vi "Laser.vi"(8 "error in (no error)":errorcluster, 10 "Notifiers":T1, 11 "All Message Queue Cluster":T2) -> (0 "error out":errorcluster)   [LabVIEW 2017]
doc: "Ce VI est la partie visualisation du Laser"
uses:
  Lib QMH/AllMessageQueue Cluster.ctl
  Lib QMH/Message Cluster.ctl
  Lib Notifier/Notifier.ctl
  Laser UI data.ctl
  PulsePickerValues.ctl
  Laser config.ctl
  FGV Laser/Action Laser.ctl
  FGV Laser/FGV Laser Data.ctl
  Lib IHM Control/Front Panel Status.ctl
  support/Status.vi
  Lib QMH/MessageQueues.lvlib
  Lib IHM Control/IHM Control.lvlib
  Lib Notifier/Notifier.lvlib
panel:
  out "Pulse Picker":dbl format="%#_3g"
  out "Power":dbl format="%#_3g"
  out "Connected":bool
  out "Status":string
  # "Laser"
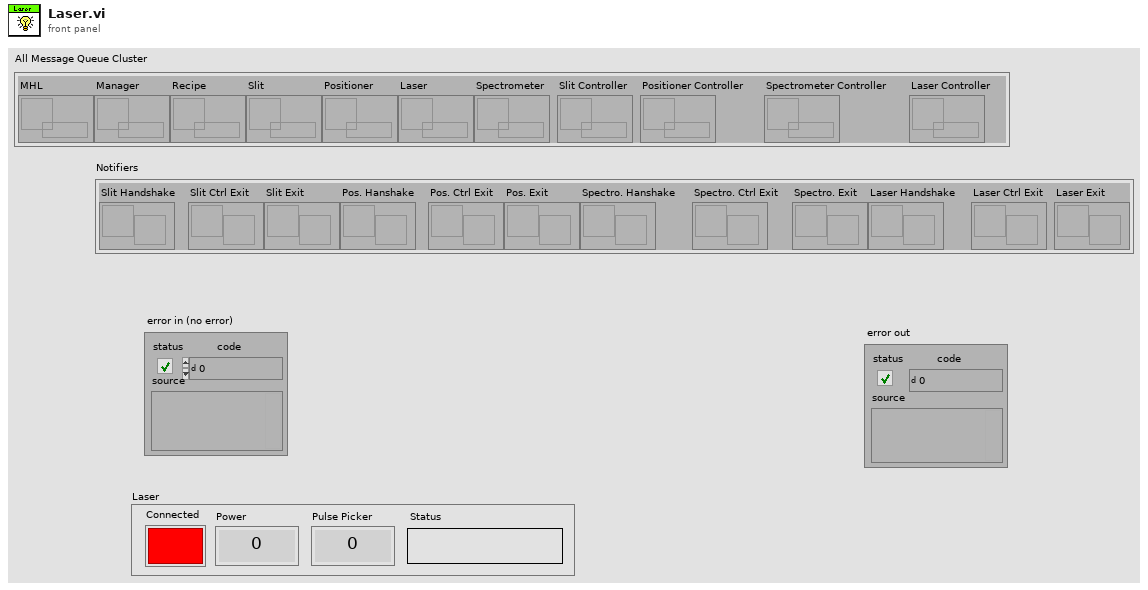
[diagram p1: front panel]
types:
  T1 = typedef "Notifier.lvlib/Notifier.ctl" = cluster{"Slit Handshake":refnum<notifier>, "Slit Ctrl Exit":refnum<notifier>, "Slit Exit":refnum<notifier>, "Pos. Hanshake":refnum<notifier>, "Pos. Ctrl Exit":refnum<notifier>, "Pos. Exit":refnum<notifier>, "Spectro. Hanshake":refnum<notifier>, "Spectro. Ctrl Exit":refnum<notifier>, "Spectro. Exit":refnum<notifier>, "Laser Handshake":refnum<notifier>, "Laser Ctrl Exit":refnum<notifier>, "Laser Exit":refnum<notifier>}
  T2 = typedef "MessageQueues.lvlib/AllMessageQueue Cluster.ctl" = cluster{"MHL":refnum<queue>, "Manager":refnum<queue>, "Recipe":refnum<queue>, "Slit":refnum<queue>, "Positioner":refnum<queue>, "Laser":refnum<queue>, "Spectrometer":refnum<queue>, "Slit Controller":refnum<queue>, "Positioner Controller":refnum<queue>, "Spectrometer Controller":refnum<queue>, "Laser Controller":refnum<queue>}
  T3 = typedef "FGV Laser Data.ctl" = cluster{"ONLINE":bool, "Power":dbl, "VISA resource name out":refnum<visa-resource-name>, "Time Out":dbl, "Status":string, "Read Count":u32, "On/OFF":bool, "Pulse Picker Set":T4}
  T4 = typedef "PulsePickerValues.ctl" = u16
  T5 = typedef "Action Laser.ctl" = enum16{"Initialize", "Connect", "Disconnect", "Set Power", "Get Power", "Set Pulse Picker", "Get Pulse Picker", "Laser ON", "Laser OFF", "Read Visa"}
  T6 = typedef "IHM Control.lvlib/Front Panel Status.ctl" = enum16{"Initialisation", "Enable Slit", "Enable Positionner", "Enable Spectrometer", "Enable Laser", "Disable Slit", "Disable Positionner", "Disable Spectrometer", "Disable Laser"}
  T7 = typedef "Laser config.ctl" = cluster{"VISA resource name":refnum<visa-resource-name>}
  T8 = typedef "Laser UI data.ctl" = cluster{"Connected":bool, "Status":string, "Power":dbl, "Pulse Picker Set":T4}
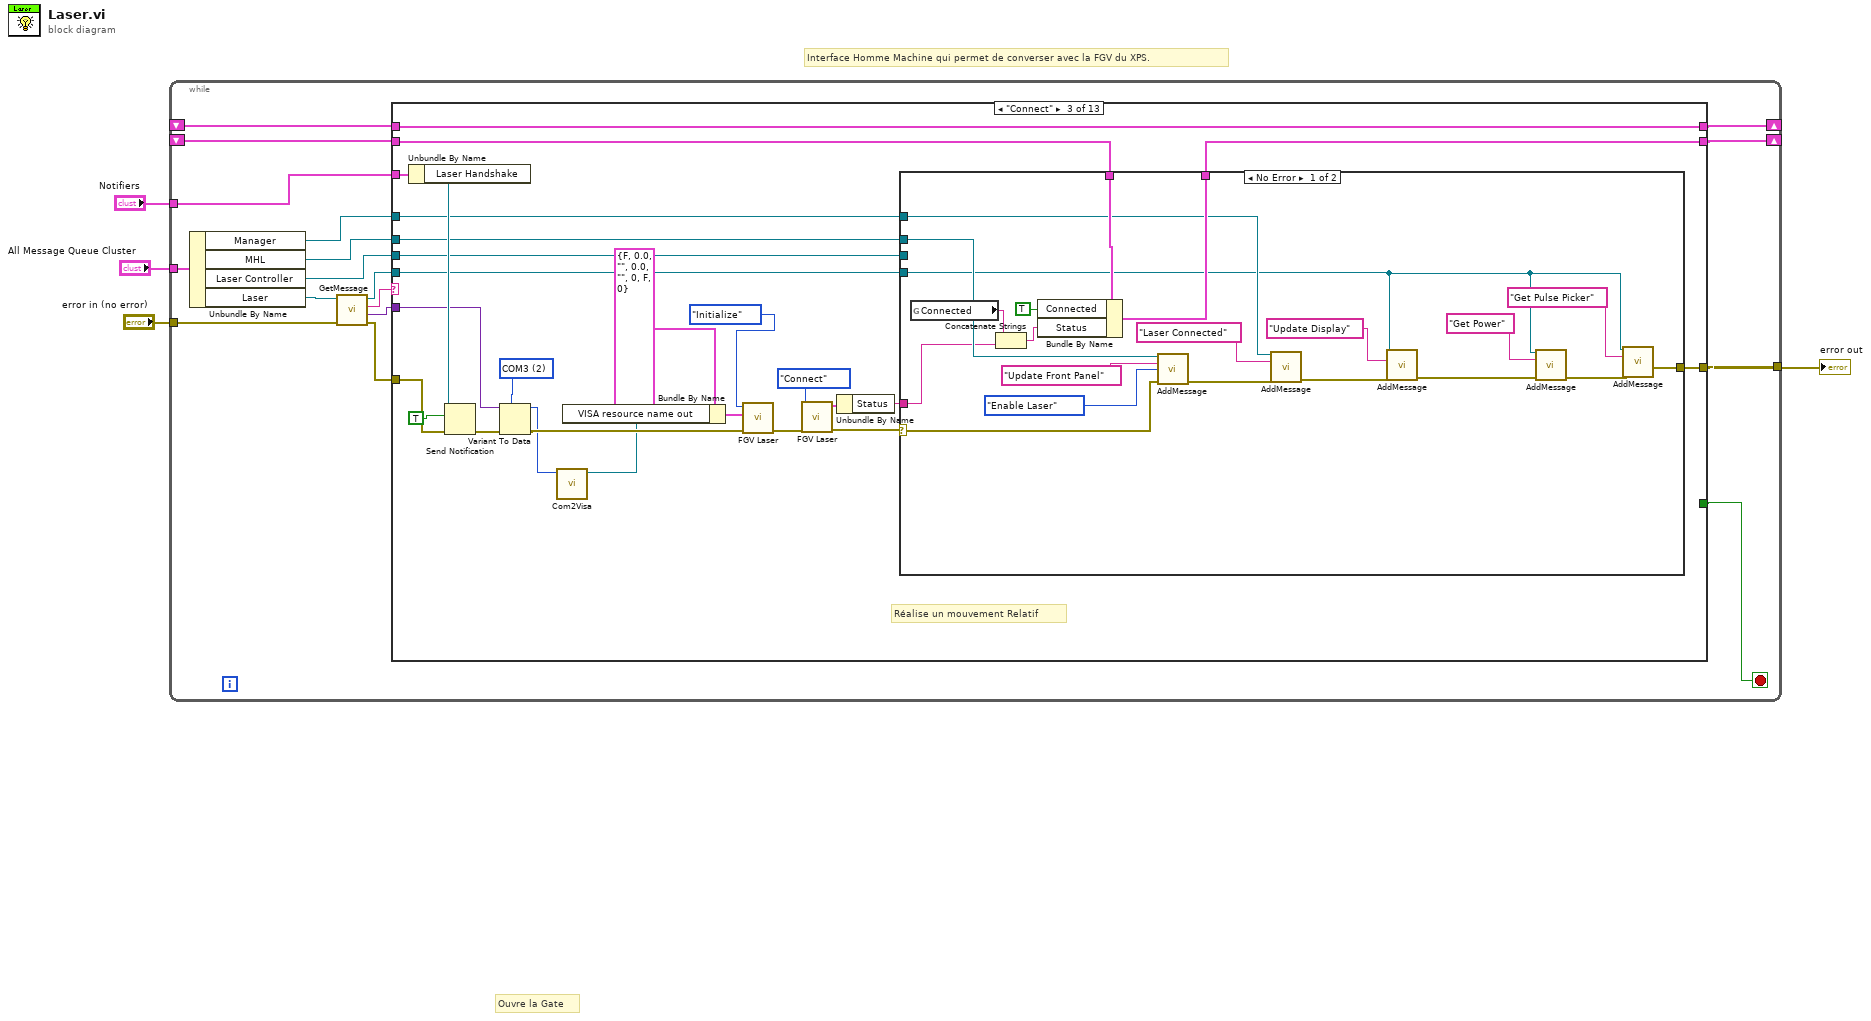
[diagram p0: block diagram]
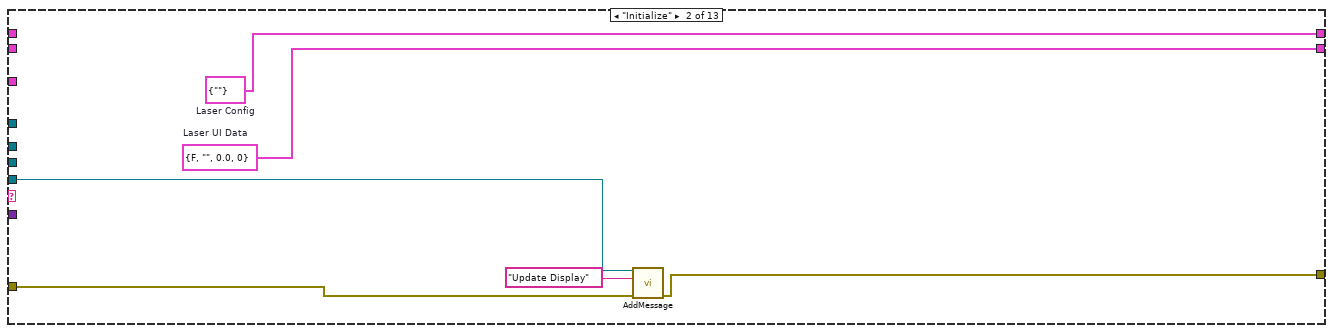
[diagram p3: hidden frame]
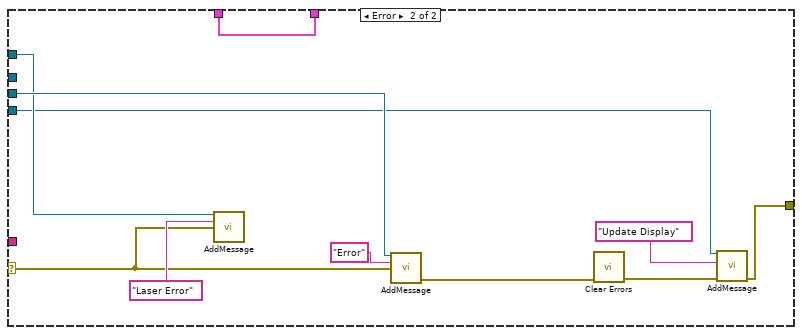
[diagram p4: hidden frame]
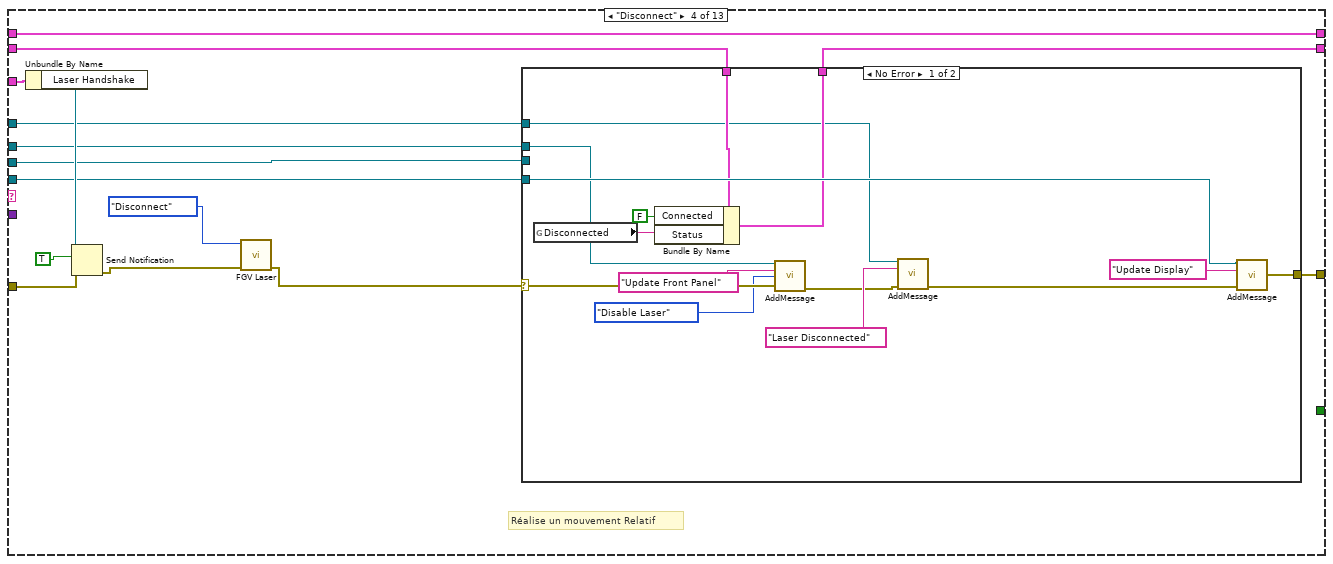
[diagram p5: hidden frame]
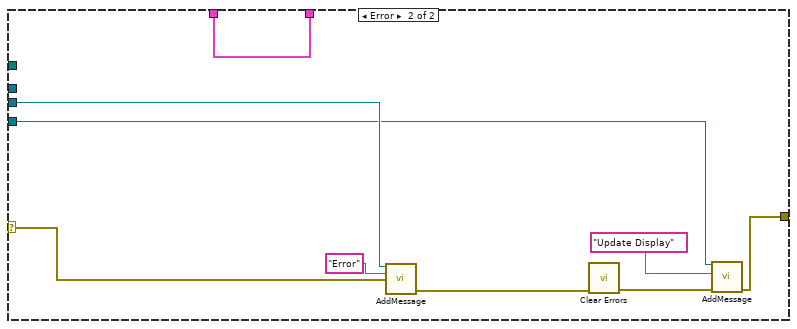
[diagram p6: hidden frame]
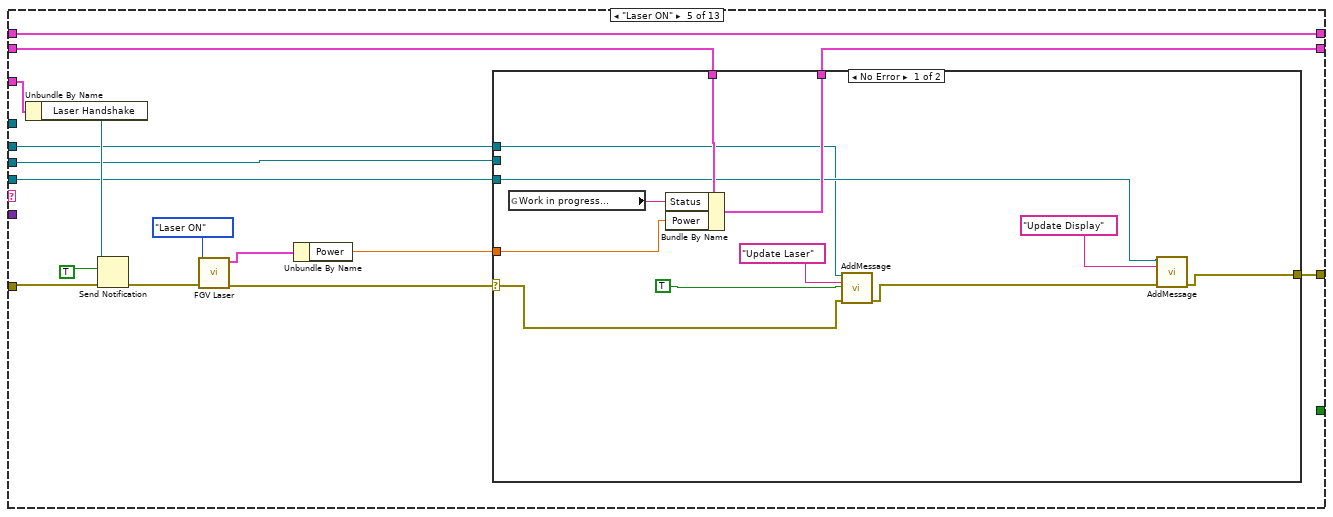
[diagram p7: hidden frame]
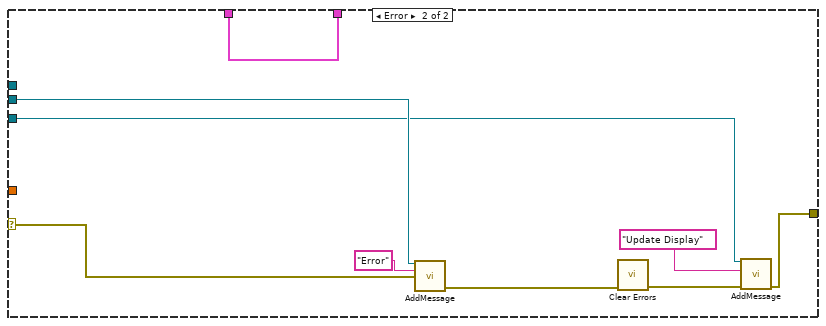
[diagram p8: hidden frame]
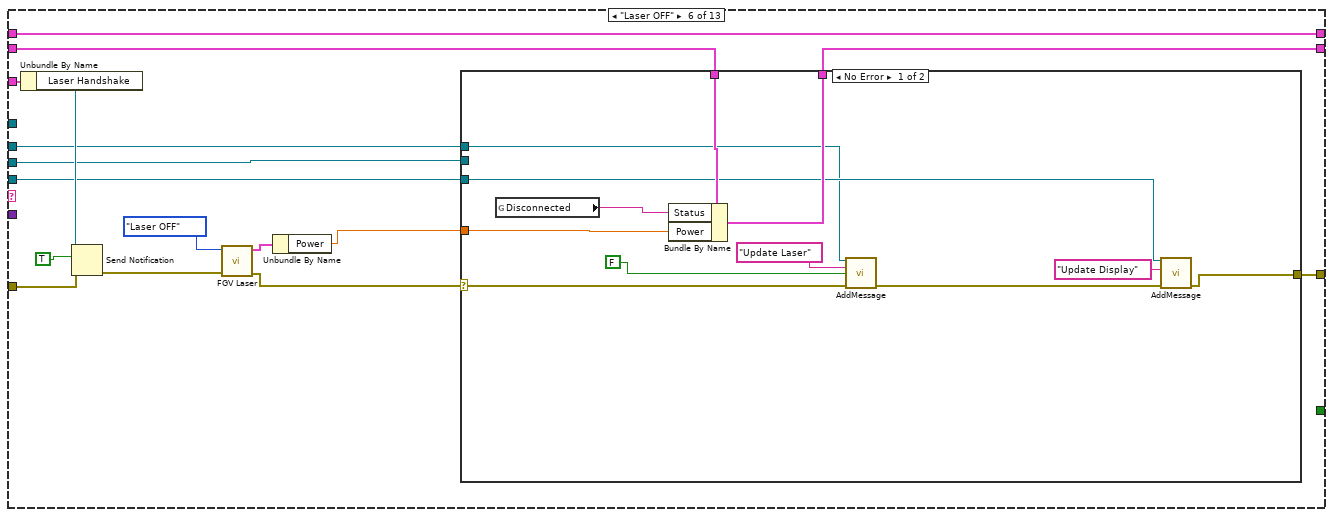
[diagram p9: hidden frame]
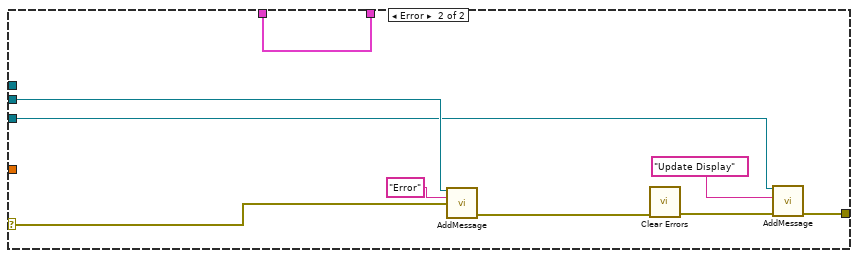
[diagram p10: hidden frame]
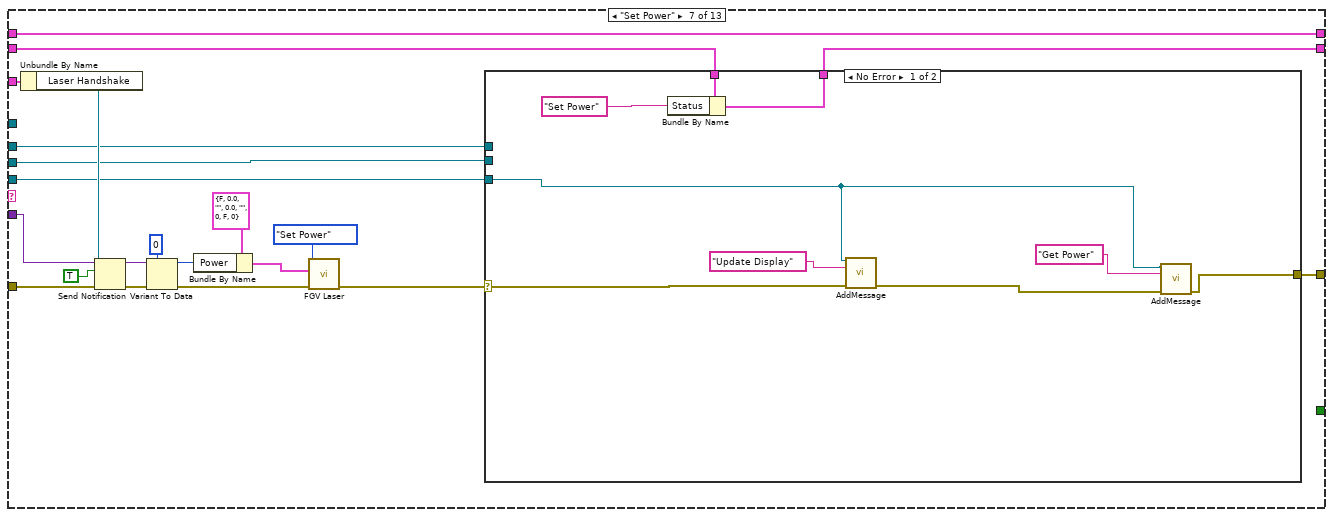
[diagram p11: hidden frame]
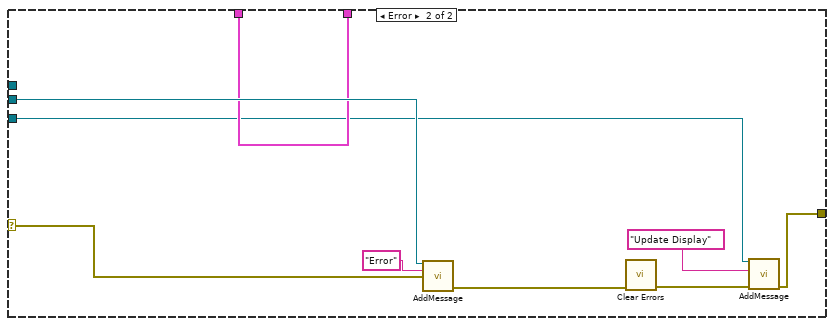
[diagram p12: hidden frame]
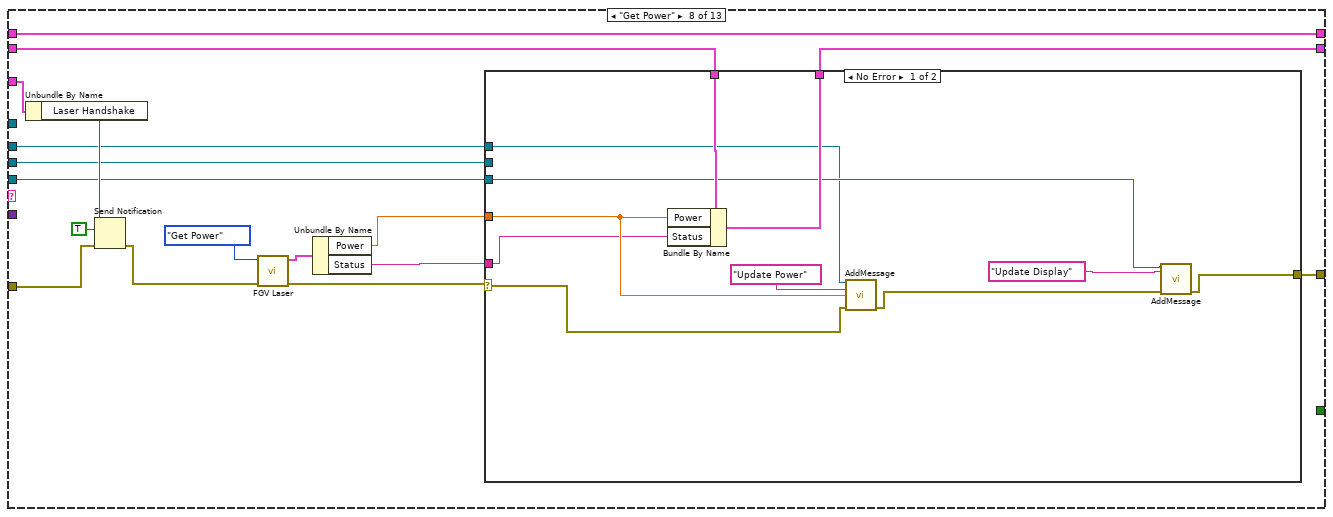
[diagram p13: hidden frame]
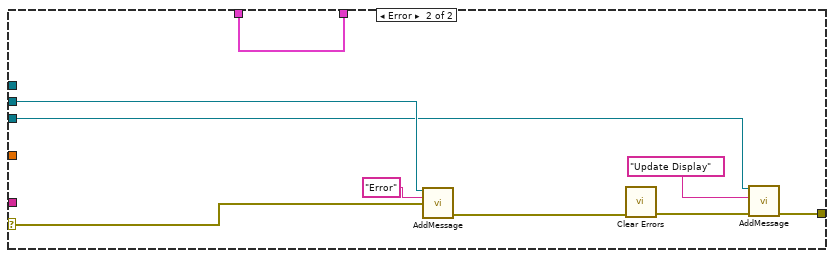
[diagram p14: hidden frame]
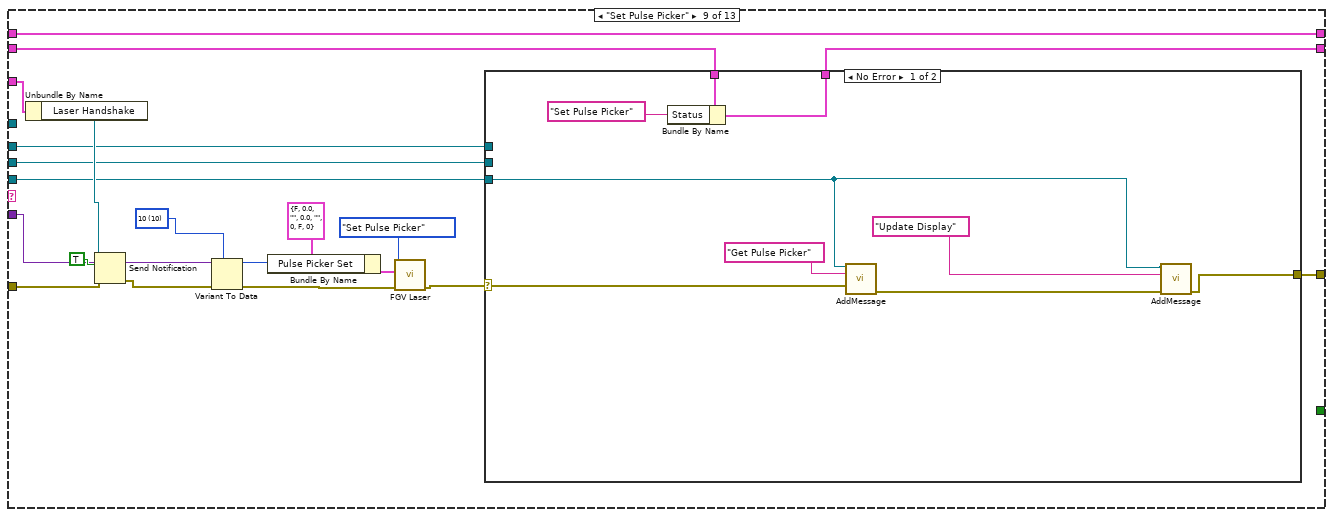
[diagram p15: hidden frame]
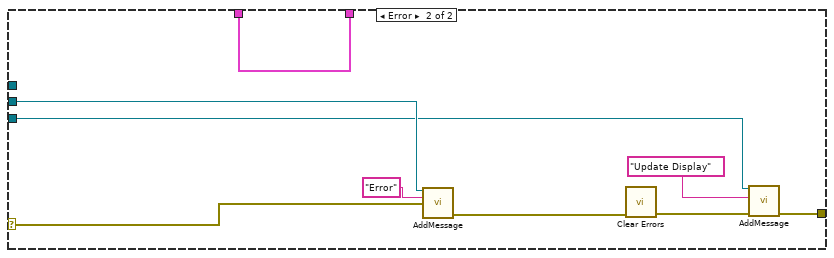
[diagram p16: hidden frame]
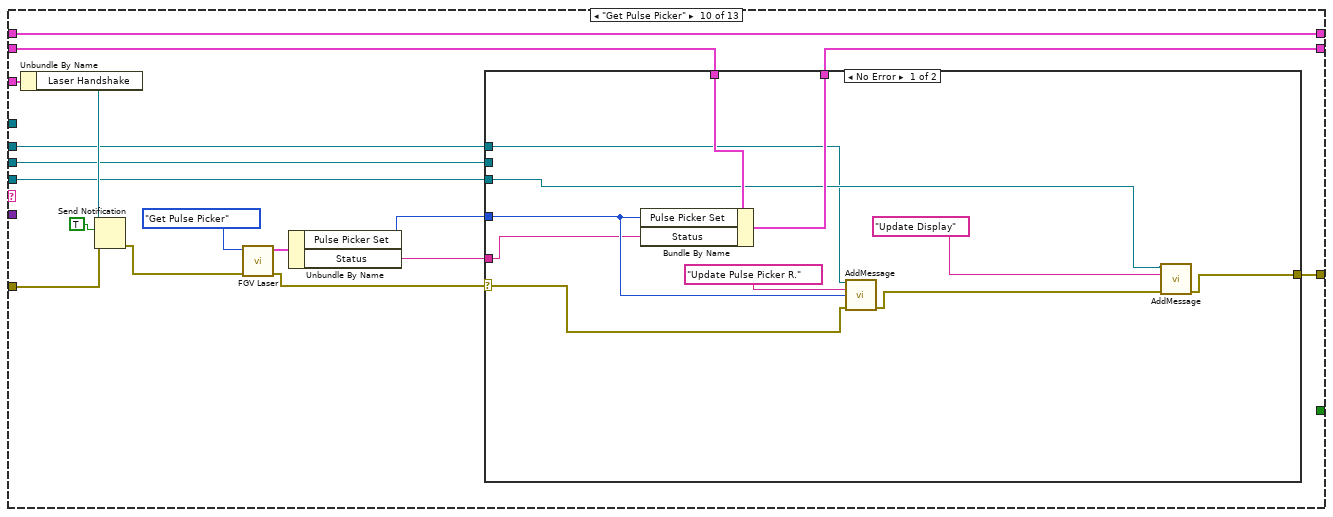
[diagram p17: hidden frame]
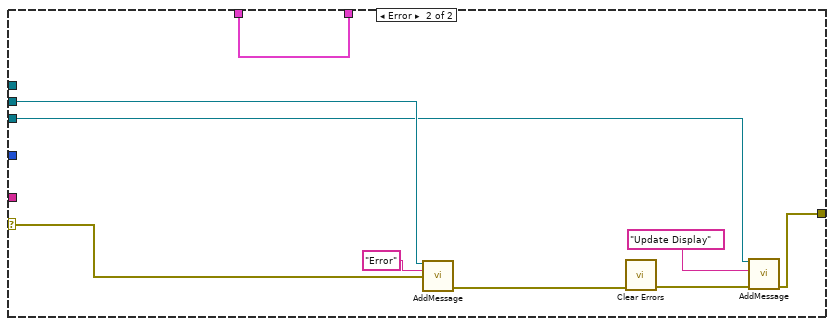
[diagram p18: hidden frame]
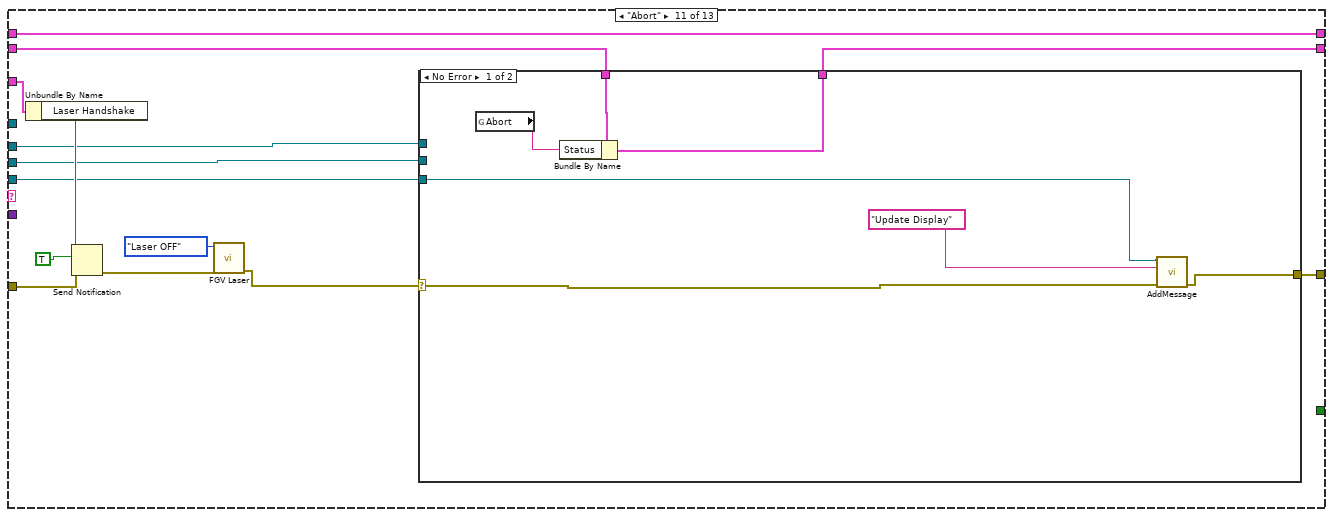
[diagram p19: hidden frame]
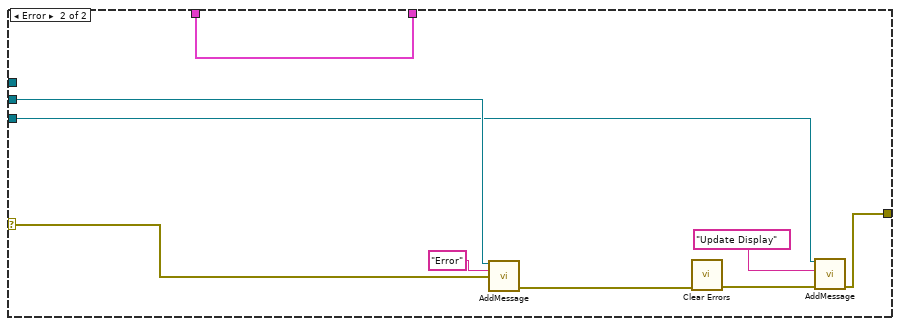
[diagram p20: hidden frame]
diagram:
  # "Interface Homme Machine qui permet de converser avec la FGV du XPS."
  # "Ouvre la Gate"
  n1 = while {
    tunnel: "All Message Queue Cluster" -> [w19]
    tunnel: "Notifiers" -> [w12]
    tunnel: "error in (no error)" -> [w20]
    tunnel: [w14] -> w1
    shift-right: [w16] -> _
    shift-left: _ -> [w18]
    shift-right: [w15] -> _
    shift-left: _ -> [w17]
    stop <- w13 stop-if-true
    n2 = Unbundle By Name(w19) -> ("Manager"=w11:refnum<queue>, "MHL"=w10:refnum<queue>, "Laser Controller"=w9:refnum<queue>, "Laser"=w21:refnum<queue>)
    n3 = call "GetMessage.vi"("entrée d'erreur"=w20, "Message queue"=w21) -> ("sortie d'erreur"=w7:errorcluster, "Data"=w6:variant, "Message"=w5:string, "Dup Message Queue"=w8:refnum<queue>)  [unwired: 6 in]
    n4 = case shown="\"Connect\"" w5 {
      tunnel: w12 -> [_ _ w54 w101 w141 w178 w219 w254 w294 w329 w363 _ w398]
      tunnel: w8 -> [_ w27 w53 w100 w140 w177 w218 w253 w293 w328 w362 _ w392]
      tunnel: w6 -> [_ _ w43 _ _ _ w211 _ w286 _ _ _ _]
      tunnel: w7 -> [w24 w29 w47 w94 w135 w172 w209 w246 w285 w321 w357 w387 w393]
      tunnel: [w24 w28 w52 w99 w139 w176 w217 w252 w292 w327 w361 w387 w395] -> w14
      tunnel: w9 -> [_ _ w51 w98 w138 w175 w216 w251 w291 w326 w360 _ _]
      tunnel: [_ _ _ _ _ _ _ _ _ _ _ _ TRUE] -> w13
      tunnel: w18 -> [w23 _ w50 w97 w137 w174 w215 w250 w290 w325 w359 w388 w394]
      tunnel: [w23 w26 w50 w97 w137 w174 w215 w250 w290 w325 w359 w388 w394] -> w16
      tunnel: w17 -> [w22 _ w49 w96 w133 w170 w212 w247 w287 w322 w355 w386 w391]
      tunnel: [w22 w25 w48 w95 w136 w173 w214 w249 w289 w324 w358 w386 w391] -> w15
      tunnel: w10 -> [_ _ w46 w93 w134 w171 w213 w248 w288 w323 w356 _ _]
      tunnel: w11 -> [_ _ w45 w92 _ _ _ _ _ _ _ _ _]
      frame Default {
        # "ne fait rien si le message dépilé n'existe pas"
      }
      frame "Initialize" {
        w26 = T7 {"VISA resource name"=""}  # Laser Config
        w25 = T8 {"Connected"=FALSE, "Status"="", "Power"=0.0, "Pulse Picker Set"=0}  # Laser UI Data
        n5 = call "AddMessage.vi"("Message queue"=w27, "Message"="Update Display", "entrée d'erreur (pas d'erreur)"=w29) -> ("error out"=w28:errorcluster)  [unwired: 11 in, 1 out]
      }
      frame "Connect" {
        w33 = 2 items=["COM1", "COM2", "COM3", "COM4", "COM5", "COM6", "COM7", "COM8", "COM9", "COM10", "COM11", "COM12", "COM13", "COM14", "COM15", "COM16", "COM17", "COM18", "COM19", "COM20", "COM21", "COM22", "COM23", "COM24", "COM25", "COM26", "COM27", "COM28", "COM29", "COM30"] ("Portnumber")
        # "Réalise un mouvement Relatif"
        n6 = Unbundle By Name(w54) -> ("Laser Handshake"=w56:refnum<notifier>)
        n7 = Send Notification(notification=TRUE, notifier=w56, error in (no error)=w47) -> (error out=w44:errorcluster)  [unwired: 1 out]
        n8 = Variant To Data(error in=w44, type=w33, Variant=w43) -> (data=w32:i32, error out=w37:errorcluster)
        n9 = call "Com2Visa.vi"("Portnumber"=w32) -> ("VISA Refnum out"=w31:refnum<visa-resource-name>)  [unwired: 10 in]
        n10 = Bundle By Name(cluster=T3 {"ONLINE"=FALSE, "Power"=0.0, "VISA resource name out"="", "Time Out"=0.0, "Status"="", "Read Count"=0, "On/OFF"=FALSE, "Pulse Picker Set"=0} ("FGV Laser Data In"), "VISA resource name out"=w31) -> (w38:T3)
        n11 = call "FGV Laser.vi"("error in (no error)"=w37, "FGV Laser Data In"=w38, "Action"=Action_Laser."Initialize") -> ("error out"=w40:errorcluster)  [unwired: 7 in, 1 out]
        n12 = call "FGV Laser.vi"("error in (no error)"=w40, "Action"=Action_Laser."Connect") -> ("error out"=w36:errorcluster, "FGV Laser Data Out"=w35:T3)  [unwired: 8 in]
        n13 = Unbundle By Name(w35) -> ("Status"=w34:string)
        n14 = case shown="No Error" w36 {
          selector: w36 -> [w73 w79]
          tunnel: w53 -> [w58 w78]
          tunnel: [w60 w84] -> w52
          tunnel: w51 -> [_ w83]
          tunnel: w49 -> [w76 w82]
          tunnel: [w75 w82] -> w48
          tunnel: w46 -> [w72 _]
          tunnel: w45 -> [w67 w80]
          tunnel: w34 -> [w63 _]
          frame No Error {
            n15 = global read "Status.vi" "Connected"() -> (w65:string)
            n16 = Concatenate Strings(w65, w63) -> (w64:string)
            n17 = Bundle By Name(cluster=w76, "Connected"=TRUE, "Status"=w64) -> (w75:T8)
            n18 = call "AddMessage.vi"("Message queue"=w72, "Message"="Update Front Panel", "Data"=Front_Panel_Status."Enable Laser" ("Front Panel status"), "entrée d'erreur (pas d'erreur)"=w73) -> ("error out"=w69:errorcluster)  [unwired: 10 in, 1 out]
            n19 = call "AddMessage.vi"("Message queue"=w67, "Message"="Laser Connected", "entrée d'erreur (pas d'erreur)"=w69) -> ("error out"=w68:errorcluster)  [unwired: 11 in, 1 out]
            n20 = call "AddMessage.vi"("Message queue"=w58, "Message"="Update Display", "entrée d'erreur (pas d'erreur)"=w68) -> ("error out"=w62:errorcluster)  [unwired: 11 in, 1 out]
            n21 = call "AddMessage.vi"("Message queue"=w58, "Message"="Get Power", "entrée d'erreur (pas d'erreur)"=w62) -> ("error out"=w61:errorcluster)  [unwired: 11 in, 1 out]
            n22 = call "AddMessage.vi"("Message queue"=w58, "Message"="Get Pulse Picker", "entrée d'erreur (pas d'erreur)"=w61) -> ("error out"=w60:errorcluster)  [unwired: 11 in, 1 out]
          }
          frame Error {
            n23 = call "AddMessage.vi"("Message queue"=w80, "Message"="Laser Error", "Data"=w79) -> ()  [unwired: 11 in, 2 out]
            n24 = call "AddMessage.vi"("Message queue"=w83, "Message"="Error", "Data"=w79) -> ("error out"=w87:errorcluster)  [unwired: 11 in, 1 out]
            n25 = call <vilib>:"Clear Errors.vi"("error in (no error)"=w87) -> ("error out"=w85:errorcluster)  [unwired: 5 in, 1 out]
            n26 = call "AddMessage.vi"("Message queue"=w78, "Message"="Update Display", "entrée d'erreur (pas d'erreur)"=w85) -> ("error out"=w84:errorcluster)  [unwired: 11 in, 1 out]
          }
        }
      }
      frame "Disconnect" {
        # "Réalise un mouvement Relatif"
        n27 = Unbundle By Name(w101) -> ("Laser Handshake"=w103:refnum<notifier>)
        n28 = Send Notification(notification=TRUE, notifier=w103, error in (no error)=w94) -> (error out=w91:errorcluster)  [unwired: 1 out]
        n29 = call "FGV Laser.vi"("error in (no error)"=w91, "Action"=Action_Laser."Disconnect") -> ("error out"=w90:errorcluster)  [unwired: 8 in, 1 out]
        n30 = case shown="No Error" w90 {
          selector: w90 -> [w112 w122]
          tunnel: w100 -> [w118 w119]
          tunnel: [w116 w123] -> w99
          tunnel: w98 -> [_ w121]
          tunnel: w96 -> [w115 w120]
          tunnel: [w114 w120] -> w95
          tunnel: w93 -> [w111 _]
          tunnel: w92 -> [w105 _]
          frame No Error {
            n31 = global read "Status.vi" "Disconnected"() -> (w104:string)
            n32 = Bundle By Name(cluster=w115, "Connected"=FALSE, "Status"=w104) -> (w114:T8)
            n33 = call "AddMessage.vi"("Message queue"=w111, "Message"="Update Front Panel", "Data"=Front_Panel_Status."Disable Laser" ("Front Panel status"), "entrée d'erreur (pas d'erreur)"=w112) -> ("error out"=w107:errorcluster)  [unwired: 10 in, 1 out]
            n34 = call "AddMessage.vi"("Message queue"=w105, "Message"="Laser Disconnected", "entrée d'erreur (pas d'erreur)"=w107) -> ("error out"=w106:errorcluster)  [unwired: 11 in, 1 out]
            n35 = call "AddMessage.vi"("Message queue"=w118, "Message"="Update Display", "entrée d'erreur (pas d'erreur)"=w106) -> ("error out"=w116:errorcluster)  [unwired: 11 in, 1 out]
          }
          frame Error {
            n36 = call "AddMessage.vi"("Message queue"=w121, "Message"="Error", "Data"=w122) -> ("error out"=w126:errorcluster)  [unwired: 11 in, 1 out]
            n37 = call <vilib>:"Clear Errors.vi"("error in (no error)"=w126) -> ("error out"=w124:errorcluster)  [unwired: 5 in, 1 out]
            n38 = call "AddMessage.vi"("Message queue"=w119, "Message"="Update Display", "entrée d'erreur (pas d'erreur)"=w124) -> ("error out"=w123:errorcluster)  [unwired: 11 in, 1 out]
          }
        }
      }
      frame "Laser ON" {
        n39 = Unbundle By Name(w141) -> ("Laser Handshake"=w143:refnum<notifier>)
        n40 = Send Notification(notification=TRUE, notifier=w143, error in (no error)=w135) -> (error out=w132:errorcluster)  [unwired: 1 out]
        n41 = call "FGV Laser.vi"("error in (no error)"=w132, "Action"=Action_Laser."Laser ON") -> ("error out"=w131:errorcluster, "FGV Laser Data Out"=w129:T3)  [unwired: 8 in]
        n42 = Unbundle By Name(w129) -> ("Power"=w128:dbl)
        n43 = case shown="No Error" w131 {
          selector: w131 -> [w151 w159]
          tunnel: w140 -> [w152 w156]
          tunnel: [w146 w160] -> w139
          tunnel: w138 -> [_ w158]
          tunnel: w133 -> [w154 w157]
          tunnel: [w153 w157] -> w136
          tunnel: w134 -> [w149 _]
          tunnel: w128 -> [w145 _]
          frame No Error {
            n44 = global read "Status.vi" "Work in progress..."() -> (w147:string)
            n45 = Bundle By Name(cluster=w154, "Status"=w147, "Power"=w145) -> (w153:T8)
            n46 = call "AddMessage.vi"("Message queue"=w149, "Message"="Update Laser", "Data"=TRUE, "entrée d'erreur (pas d'erreur)"=w151) -> ("error out"=w150:errorcluster)  [unwired: 10 in, 1 out]
            n47 = call "AddMessage.vi"("Message queue"=w152, "Message"="Update Display", "entrée d'erreur (pas d'erreur)"=w150) -> ("error out"=w146:errorcluster)  [unwired: 11 in, 1 out]
          }
          frame Error {
            n48 = call "AddMessage.vi"("Message queue"=w158, "Message"="Error", "Data"=w159) -> ("error out"=w163:errorcluster)  [unwired: 11 in, 1 out]
            n49 = call <vilib>:"Clear Errors.vi"("error in (no error)"=w163) -> ("error out"=w161:errorcluster)  [unwired: 5 in, 1 out]
            n50 = call "AddMessage.vi"("Message queue"=w156, "Message"="Update Display", "entrée d'erreur (pas d'erreur)"=w161) -> ("error out"=w160:errorcluster)  [unwired: 11 in, 1 out]
          }
        }
      }
      frame "Laser OFF" {
        n51 = Unbundle By Name(w178) -> ("Laser Handshake"=w180:refnum<notifier>)
        n52 = Send Notification(notification=TRUE, notifier=w180, error in (no error)=w172) -> (error out=w169:errorcluster)  [unwired: 1 out]
        n53 = call "FGV Laser.vi"("error in (no error)"=w169, "Action"=Action_Laser."Laser OFF") -> ("error out"=w168:errorcluster, "FGV Laser Data Out"=w166:T3)  [unwired: 8 in]
        n54 = Unbundle By Name(w166) -> ("Power"=w165:dbl)
        n55 = case shown="No Error" w168 {
          selector: w168 -> [w183 w196]
          tunnel: w177 -> [w186 w193]
          tunnel: [w184 w197] -> w176
          tunnel: w175 -> [_ w195]
          tunnel: w170 -> [w188 w194]
          tunnel: [w187 w194] -> w173
          tunnel: w171 -> [w185 _]
          tunnel: w165 -> [w182 _]
          frame No Error {
            n56 = global read "Status.vi" "Disconnected"() -> (w189:string)
            n57 = Bundle By Name(cluster=w188, "Status"=w189, "Power"=w182) -> (w187:T8)
            n58 = call "AddMessage.vi"("Message queue"=w185, "Message"="Update Laser", "Data"=FALSE, "entrée d'erreur (pas d'erreur)"=w183) -> ("error out"=w191:errorcluster)  [unwired: 10 in, 1 out]
            n59 = call "AddMessage.vi"("Message queue"=w186, "Message"="Update Display", "entrée d'erreur (pas d'erreur)"=w191) -> ("error out"=w184:errorcluster)  [unwired: 11 in, 1 out]
          }
          frame Error {
            n60 = call "AddMessage.vi"("Message queue"=w195, "Message"="Error", "Data"=w196) -> ("error out"=w200:errorcluster)  [unwired: 11 in, 1 out]
            n61 = call <vilib>:"Clear Errors.vi"("error in (no error)"=w200) -> ("error out"=w198:errorcluster)  [unwired: 5 in, 1 out]
            n62 = call "AddMessage.vi"("Message queue"=w193, "Message"="Update Display", "entrée d'erreur (pas d'erreur)"=w198) -> ("error out"=w197:errorcluster)  [unwired: 11 in, 1 out]
          }
        }
      }
      frame "Set Power" {
        n63 = Unbundle By Name(w219) -> ("Laser Handshake"=w221:refnum<notifier>)
        n64 = Send Notification(notification=TRUE, notifier=w221, error in (no error)=w209) -> (error out=w208:errorcluster)  [unwired: 1 out]
        n65 = Variant To Data(error in=w208, type=u16 0, Variant=w211) -> (data=w206:u16, error out=w204:errorcluster)
        n66 = Bundle By Name(cluster=T3 {"ONLINE"=FALSE, "Power"=0.0, "VISA resource name out"="", "Time Out"=0.0, "Status"="", "Read Count"=0, "On/OFF"=FALSE, "Pulse Picker Set"=0} ("FGV Laser Data In"), "Power"=w206) -> (w205:T3)
        n67 = call "FGV Laser.vi"("error in (no error)"=w204, "FGV Laser Data In"=w205, "Action"=Action_Laser."Set Power") -> ("error out"=w203:errorcluster)  [unwired: 7 in, 1 out]
        n68 = case shown="No Error" w203 {
          selector: w203 -> [w227 w234]
          tunnel: w218 -> [w224 w231]
          tunnel: [w226 w235] -> w217
          tunnel: w216 -> [_ w233]
          tunnel: w212 -> [w229 w232]
          tunnel: [w228 w232] -> w214
          tunnel: w213 -> [_ _]
          frame No Error {
            n69 = Bundle By Name(cluster=w229, "Status"="Set Power") -> (w228:T8)
            n70 = call "AddMessage.vi"("Message queue"=w224, "Message"="Update Display", "entrée d'erreur (pas d'erreur)"=w227) -> ("error out"=w230:errorcluster)  [unwired: 11 in, 1 out]
            n71 = call "AddMessage.vi"("Message queue"=w224, "Message"="Get Power", "entrée d'erreur (pas d'erreur)"=w230) -> ("error out"=w226:errorcluster)  [unwired: 11 in, 1 out]
          }
          frame Error {
            n72 = call "AddMessage.vi"("Message queue"=w233, "Message"="Error", "Data"=w234) -> ("error out"=w238:errorcluster)  [unwired: 11 in, 1 out]
            n73 = call <vilib>:"Clear Errors.vi"("error in (no error)"=w238) -> ("error out"=w236:errorcluster)  [unwired: 5 in, 1 out]
            n74 = call "AddMessage.vi"("Message queue"=w231, "Message"="Update Display", "entrée d'erreur (pas d'erreur)"=w236) -> ("error out"=w235:errorcluster)  [unwired: 11 in, 1 out]
          }
        }
      }
      frame "Get Power" {
        n75 = Unbundle By Name(w254) -> ("Laser Handshake"=w256:refnum<notifier>)
        n76 = Send Notification(notification=TRUE, notifier=w256, error in (no error)=w246) -> (error out=w245:errorcluster)  [unwired: 1 out]
        n77 = call "FGV Laser.vi"("error in (no error)"=w245, "Action"=Action_Laser."Get Power") -> ("error out"=w244:errorcluster, "FGV Laser Data Out"=w242:T3)  [unwired: 8 in]
        n78 = Unbundle By Name(w242) -> ("Power"=w241:dbl, "Status"=w240:string)
        n79 = case shown="No Error" w244 {
          selector: w244 -> [w262 w271]
          tunnel: w253 -> [w260 w268]
          tunnel: [w261 w272] -> w252
          tunnel: w251 -> [_ w270]
          tunnel: w247 -> [w264 w269]
          tunnel: [w263 w269] -> w249
          tunnel: w248 -> [w259 _]
          tunnel: w241 -> [w258 _]
          tunnel: w240 -> [w257 _]
          frame No Error {
            n80 = Bundle By Name(cluster=w264, "Power"=w258, "Status"=w257) -> (w263:T8)
            n81 = call "AddMessage.vi"("Message queue"=w259, "Message"="Update Power", "Data"=w258, "entrée d'erreur (pas d'erreur)"=w262) -> ("error out"=w266:errorcluster)  [unwired: 10 in, 1 out]
            n82 = call "AddMessage.vi"("Message queue"=w260, "Message"="Update Display", "entrée d'erreur (pas d'erreur)"=w266) -> ("error out"=w261:errorcluster)  [unwired: 11 in, 1 out]
          }
          frame Error {
            n83 = call "AddMessage.vi"("Message queue"=w270, "Message"="Error", "Data"=w271) -> ("error out"=w275:errorcluster)  [unwired: 11 in, 1 out]
            n84 = call <vilib>:"Clear Errors.vi"("error in (no error)"=w275) -> ("error out"=w273:errorcluster)  [unwired: 5 in, 1 out]
            n85 = call "AddMessage.vi"("Message queue"=w268, "Message"="Update Display", "entrée d'erreur (pas d'erreur)"=w273) -> ("error out"=w272:errorcluster)  [unwired: 11 in, 1 out]
          }
        }
      }
      frame "Set Pulse Picker" {
        w277 = T4 10 items=["80"=80, "40"=40, "20"=20, "10"=10, "0"=0] ("Pulse Picker Set")
        n86 = Unbundle By Name(w294) -> ("Laser Handshake"=w296:refnum<notifier>)
        n87 = Send Notification(notification=TRUE, notifier=w296, error in (no error)=w285) -> (error out=w284:errorcluster)  [unwired: 1 out]
        n88 = Variant To Data(error in=w284, type=w277, Variant=w286) -> (data=w278:T4, error out=w283:errorcluster)
        n89 = Bundle By Name(cluster=T3 {"ONLINE"=FALSE, "Power"=0.0, "VISA resource name out"="", "Time Out"=0.0, "Status"="", "Read Count"=0, "On/OFF"=FALSE, "Pulse Picker Set"=0} ("FGV Laser Data In"), "Pulse Picker Set"=w278) -> (w280:T3)
        n90 = call "FGV Laser.vi"("error in (no error)"=w283, "FGV Laser Data In"=w280, "Action"=Action_Laser."Set Pulse Picker") -> ("error out"=w282:errorcluster)  [unwired: 7 in, 1 out]
        n91 = case shown="No Error" w282 {
          selector: w282 -> [w300 w309]
          tunnel: w293 -> [w297 w306]
          tunnel: [w299 w310] -> w292
          tunnel: w291 -> [_ w308]
          tunnel: w287 -> [w302 w307]
          tunnel: [w301 w307] -> w289
          tunnel: w288 -> [_ _]
          frame No Error {
            n92 = Bundle By Name(cluster=w302, "Status"="Set Pulse Picker") -> (w301:T8)
            n93 = call "AddMessage.vi"("Message queue"=w297, "Message"="Get Pulse Picker", "entrée d'erreur (pas d'erreur)"=w300) -> ("error out"=w304:errorcluster)  [unwired: 11 in, 1 out]
            n94 = call "AddMessage.vi"("Message queue"=w297, "Message"="Update Display", "entrée d'erreur (pas d'erreur)"=w304) -> ("error out"=w299:errorcluster)  [unwired: 11 in, 1 out]
          }
          frame Error {
            n95 = call "AddMessage.vi"("Message queue"=w308, "Message"="Error", "Data"=w309) -> ("error out"=w313:errorcluster)  [unwired: 11 in, 1 out]
            n96 = call <vilib>:"Clear Errors.vi"("error in (no error)"=w313) -> ("error out"=w311:errorcluster)  [unwired: 5 in, 1 out]
            n97 = call "AddMessage.vi"("Message queue"=w306, "Message"="Update Display", "entrée d'erreur (pas d'erreur)"=w311) -> ("error out"=w310:errorcluster)  [unwired: 11 in, 1 out]
          }
        }
      }
      frame "Get Pulse Picker" {
        n98 = Unbundle By Name(w329) -> ("Laser Handshake"=w331:refnum<notifier>)
        n99 = Send Notification(notification=TRUE, notifier=w331, error in (no error)=w321) -> (error out=w320:errorcluster)  [unwired: 1 out]
        n100 = call "FGV Laser.vi"("error in (no error)"=w320, "Action"=Action_Laser."Get Pulse Picker") -> ("error out"=w319:errorcluster, "FGV Laser Data Out"=w317:T3)  [unwired: 8 in]
        n101 = Unbundle By Name(w317) -> ("Pulse Picker Set"=w316:T4, "Status"=w315:string)
        n102 = case shown="No Error" w319 {
          selector: w319 -> [w337 w346]
          tunnel: w328 -> [w335 w343]
          tunnel: [w336 w347] -> w327
          tunnel: w326 -> [_ w345]
          tunnel: w322 -> [w339 w344]
          tunnel: [w338 w344] -> w324
          tunnel: w323 -> [w334 _]
          tunnel: w316 -> [w333 _]
          tunnel: w315 -> [w332 _]
          frame No Error {
            n103 = Bundle By Name(cluster=w339, "Pulse Picker Set"=w333, "Status"=w332) -> (w338:T8)
            n104 = call "AddMessage.vi"("Message queue"=w334, "Message"="Update Pulse Picker R.", "Data"=w333, "entrée d'erreur (pas d'erreur)"=w337) -> ("error out"=w341:errorcluster)  [unwired: 10 in, 1 out]
            n105 = call "AddMessage.vi"("Message queue"=w335, "Message"="Update Display", "entrée d'erreur (pas d'erreur)"=w341) -> ("error out"=w336:errorcluster)  [unwired: 11 in, 1 out]
          }
          frame Error {
            n106 = call "AddMessage.vi"("Message queue"=w345, "Message"="Error", "Data"=w346) -> ("error out"=w350:errorcluster)  [unwired: 11 in, 1 out]
            n107 = call <vilib>:"Clear Errors.vi"("error in (no error)"=w350) -> ("error out"=w348:errorcluster)  [unwired: 5 in, 1 out]
            n108 = call "AddMessage.vi"("Message queue"=w343, "Message"="Update Display", "entrée d'erreur (pas d'erreur)"=w348) -> ("error out"=w347:errorcluster)  [unwired: 11 in, 1 out]
          }
        }
      }
      frame "Abort" {
        n109 = Unbundle By Name(w363) -> ("Laser Handshake"=w365:refnum<notifier>)
        n110 = Send Notification(notification=TRUE, notifier=w365, error in (no error)=w357) -> (error out=w354:errorcluster)  [unwired: 1 out]
        n111 = call "FGV Laser.vi"("error in (no error)"=w354, "Action"=Action_Laser."Laser OFF") -> ("error out"=w352:errorcluster)  [unwired: 8 in, 1 out]
        n112 = case shown="No Error" w352 {
          selector: w352 -> [w370 w376]
          tunnel: w362 -> [w371 w373]
          tunnel: [w369 w377] -> w361
          tunnel: w360 -> [_ w375]
          tunnel: w355 -> [w368 w374]
          tunnel: [w367 w374] -> w358
          tunnel: w356 -> [_ _]
          frame No Error {
            n113 = global read "Status.vi" "Abort"() -> (w366:string)
            n114 = Bundle By Name(cluster=w368, "Status"=w366) -> (w367:T8)
            n115 = call "AddMessage.vi"("Message queue"=w371, "Message"="Update Display", "entrée d'erreur (pas d'erreur)"=w370) -> ("error out"=w369:errorcluster)  [unwired: 11 in, 1 out]
          }
          frame Error {
            n116 = call "AddMessage.vi"("Message queue"=w375, "Message"="Error", "Data"=w376) -> ("error out"=w380:errorcluster)  [unwired: 11 in, 1 out]
            n117 = call <vilib>:"Clear Errors.vi"("error in (no error)"=w380) -> ("error out"=w378:errorcluster)  [unwired: 5 in, 1 out]
            n118 = call "AddMessage.vi"("Message queue"=w373, "Message"="Update Display", "entrée d'erreur (pas d'erreur)"=w378) -> ("error out"=w377:errorcluster)  [unwired: 11 in, 1 out]
          }
        }
      }
      frame "Update Display" {
        # "Met à jour les valeur Init, Status et position"
        n119 = Unbundle By Name(w386) -> ("Connected"=→"Connected":bool, "Status"=→"Status":string, "Power"=→"Power":dbl, "Pulse Picker Set"=→"Pulse Picker":T4)
      }
      frame "Exit" {
        n120 = Unbundle By Name(w398) -> ("Laser Exit"=w397:refnum<notifier>)
        n121 = Release Queue(queue=w392, error in (no error)=w393) -> (error out=w389:errorcluster)  [unwired: 1 in, 2 out]
        n122 = call <vilib>:"Clear Errors.vi"("error in (no error)"=w389) -> ("error out"=w390:errorcluster)  [unwired: 5 in, 1 out]
        n123 = Send Notification(notification=TRUE, notifier=w397, error in (no error)=w390) -> (error out=w395:errorcluster)  [unwired: 1 out]
      }
    }
  }
  "error out" <- w1
